vi "Ultrasonic Data V2015.vi"(0 "FPGA VI Reference in":refnum<k20>, 1 "error in":errorcluster) -> (2 "FPGA VI Reference Out":refnum<k20>, 3 "error out":errorcluster, 4 "Front L/R":cluster{i32, i32}, 5 "Center L/R":cluster{i32, i32})   [LabVIEW 2014]
uses:
  <vilib>/Utility/error.llb/Error Cluster From Error Code.vi
  <vilib>/rvi/errors/niLvFpgaAdjustHostInterfaceError.vi
  <vilib>/rvi/interface/nirviReadWriteControl/nirviReadWriteControl.xnode
  NiFpgaLv.dll
  <vilib>/rvi/interface/Simulation/niFpgaSimulationCallBeginRW.vi
panel:
  out "Center Right Dist":i32
  out "Center Left Dist":i32
  out "Center Right Dist (cm) 3":fxp<+,24,16>
  out "Front Left Dist (cm) 2":fxp<+,24,16>
  out "Front Right Dist (cm) 2":fxp<+,24,16>
  out "Centre Left Dist (cm) 2":fxp<+,24,16>
  out "Centre Right Dist (cm) 2":fxp<+,24,16>
  out "Front Left Dist (cm)":i32
  out "Front Right Dist (cm)":i32
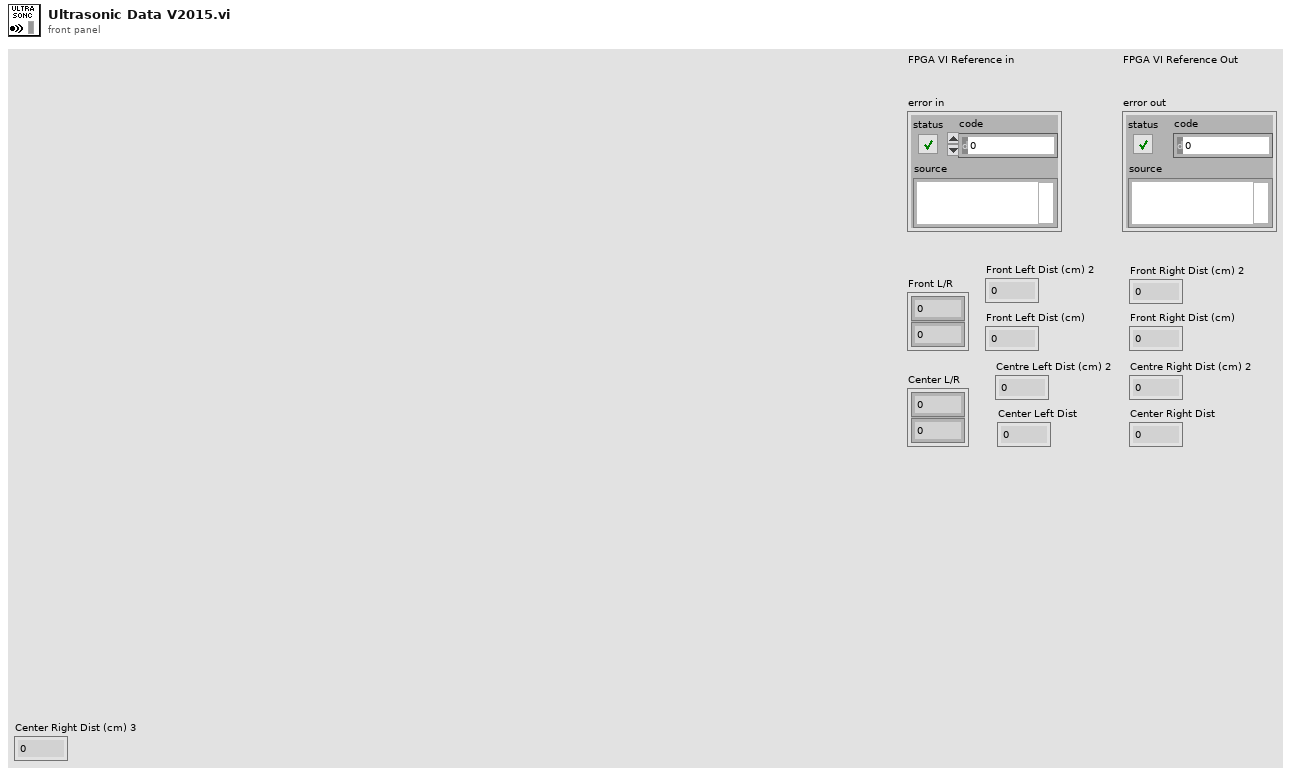
[diagram p1: front panel]
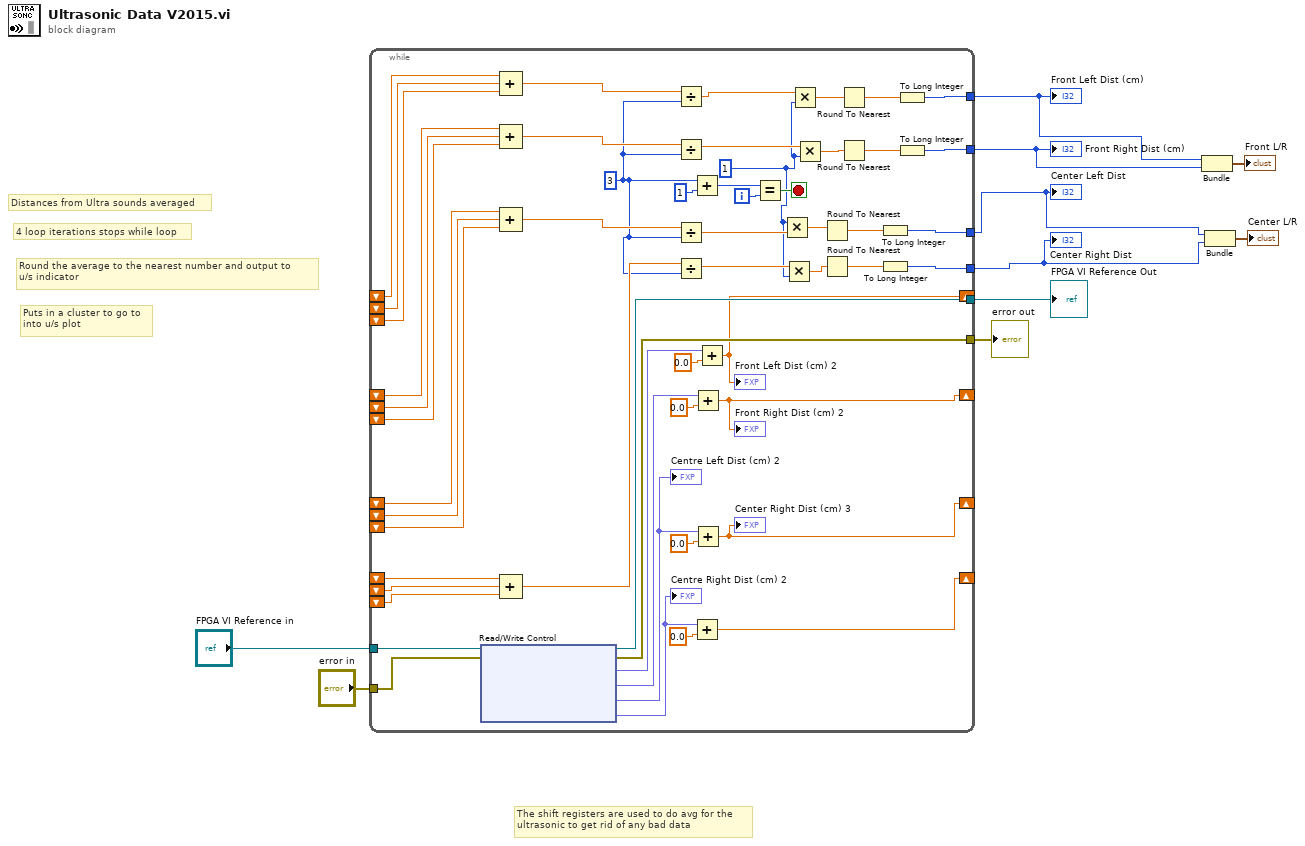
[diagram p0: block diagram]
diagram:
  # "Puts in a cluster to go to\ninto u/s plot"
  # "Round the average to the nearest number and output to \nu/s indicator"
  # "4 loop iterations stops while loop"
  # "Distances from Ultra sounds averaged"
  # "The shift registers are used to do avg for the \nultrasonic to get rid of any bad data"
  n1 = while {
    tunnel: "FPGA VI Reference in" -> [w64]
    tunnel: "error in" -> [w63]
    tunnel: [w62] -> w10
    tunnel: [w61] -> w9
    shift-right: [w40] -> _
    shift-left: _ -> [w60]
    shift-right: [w41] -> _
    shift-left: _ -> [w57]
    shift-left: _ -> [w59]
    shift-left: _ -> [w58]
    shift-left: _ -> [w56]
    shift-left: _ -> [w55]
    tunnel: [w47] -> w5
    tunnel: [w46] -> w6
    shift-right: [w37] -> _
    shift-left: _ -> [w36]
    shift-left: _ -> [w35]
    shift-left: _ -> [w34]
    tunnel: [w31] -> w3
    shift-right: [w26] -> _
    shift-left: _ -> [w25]
    shift-left: _ -> [w24]
    shift-left: _ -> [w23]
    tunnel: [w22] -> w2
    i -> [w51]
    stop <- w50 stop-if-true
    w13 = 1 ("y")
    w11 = 3 ("y")
    n2 = xnode "Read/Write Control"("FPGA VI Reference In"=w64, "error in"=w63) -> ("FPGA VI Reference Out"=w62:refnum<k20>, "error out"=w61:errorcluster, "Front Left Dist (cm)"=w45:fxp<+,24,16>, "Front Right Dist (cm)"=w42:fxp<+,24,16>, "Centre Left Dist (cm)"=w38:fxp<+,24,16>, "Centre Right Dist (cm)"=w27:fxp<+,24,16>)
    "Centre Left Dist (cm) 2" <- w38
    "Centre Right Dist (cm) 2" <- w27
    n3 = Compound Arithmetic op=ADD(w60, w59, w58) -> (w54:dbl)
    n4 = Compound Arithmetic op=ADD(w57, w56, w55) -> (w53:dbl)
    n5 = Compound Arithmetic op=ADD(w36, w35, w34) -> (w32:dbl)
    n6 = Compound Arithmetic op=ADD(w25, w24, w23) -> (w29:dbl)
    n7 = Divide(x=w54, y=w11) -> (x/y=w17:dbl)
    n8 = Divide(x=w53, y=w11) -> (x/y=w18:dbl)
    n9 = Divide(x=w32, y=w11) -> (x/y=w15:dbl)
    n10 = Divide(x=w29, y=w11) -> (x/y=w14:dbl)
    n11 = Add(x=w11, y=1) -> (x+y=w48:i32)
    n12 = Add(x=w27, y=0.0 ("x")) -> (x+y=w26:dbl)
    n13 = Add(x=w42, y=0.0 ("x")) -> (x+y=w41:dbl)
    "Front Right Dist (cm) 2" <- w41
    n14 = Add(x=w38, y=0.0 ("x")) -> (x+y=w37:dbl)
    "Center Right Dist (cm) 3" <- w37
    n15 = Add(x=w45, y=0.0 ("x")) -> (x+y=w40:dbl)
    "Front Left Dist (cm) 2" <- w40
    n16 = Equal?(x=w48, y=w51) -> (x = y?=w50:bool)
    n17 = Multiply(x=w13, y=w15) -> (x*y=w16:dbl)
    n18 = Multiply(x=w14, y=w13) -> (x*y=w12:dbl)
    n19 = Multiply(x=w17, y=w13) -> (x*y=w20:dbl)
    n20 = Multiply(x=w18, y=w13) -> (x*y=w19:dbl)
    n21 = Round To Nearest(number=w16) -> (nearest integer value=w33:dbl)
    n22 = Round To Nearest(number=w12) -> (nearest integer value=w30:dbl)
    n23 = Round To Nearest(number=w20) -> (nearest integer value=w21:dbl)
    n24 = Round To Nearest(number=w19) -> (nearest integer value=w52:dbl)
    n25 = To Long Integer(number=w33) -> (32bit integer=w31:i32)
    n26 = To Long Integer(number=w30) -> (32bit integer=w22:i32)
    n27 = To Long Integer(number=w21) -> (32bit integer=w46:i32)
    n28 = To Long Integer(number=w52) -> (32bit integer=w47:i32)
  }
  "FPGA VI Reference Out" <- w10
  "error out" <- w9
  "Front Right Dist (cm)" <- w5
  "Front Left Dist (cm)" <- w6
  "Center Left Dist" <- w3
  "Center Right Dist" <- w2
  n29 = Bundle(w6, w5) -> (→"Front L/R":cluster{i32, i32})  [unwired: 1 in]
  n30 = Bundle(w3, w2) -> (→"Center L/R":cluster{i32, i32})  [unwired: 1 in]
